vi "ERD Send Receive Example.vi"() -> ()   [LabVIEW 2016]
uses:
  type defs/ERD Read Data Out.ctl
  type defs/ERD Read Data In.ctl
  type defs/Data Type.ctl
  type defs/ERD Write Data In.ctl
  type defs/Source_Destination.ctl
  <vilib>/Utility/file.llb/Write To Spreadsheet File (string).vi
  library/GEA2_Toolkit.lvlib
panel:
  out "Continouous":T1[](array[typedef]) {"ERD Number" format="%.0x"}
  out "Raw Data Out":string
  in  "Write ERD List":T2[](array[typedef]) {"ERD Number" format="%.0x"}
  in  "Send ERD":bool
  in  "ERD to Read":T4[](array[typedef])=[{"ERD Number"=16499, "Data Type"=enum."string"}] {"ERD Number" format="%.0x"}
  out "Output Data Read":T1[](array[typedef]) {"ERD Number" format="%.0x"}
  in  "Read ERD":bool
  in  "Path":path
  in  "Board Index":i32
  in  "stop":bool
  # "HEWH Wifi Module\n0x600F - 01 Off\n0x600F - 00 On"
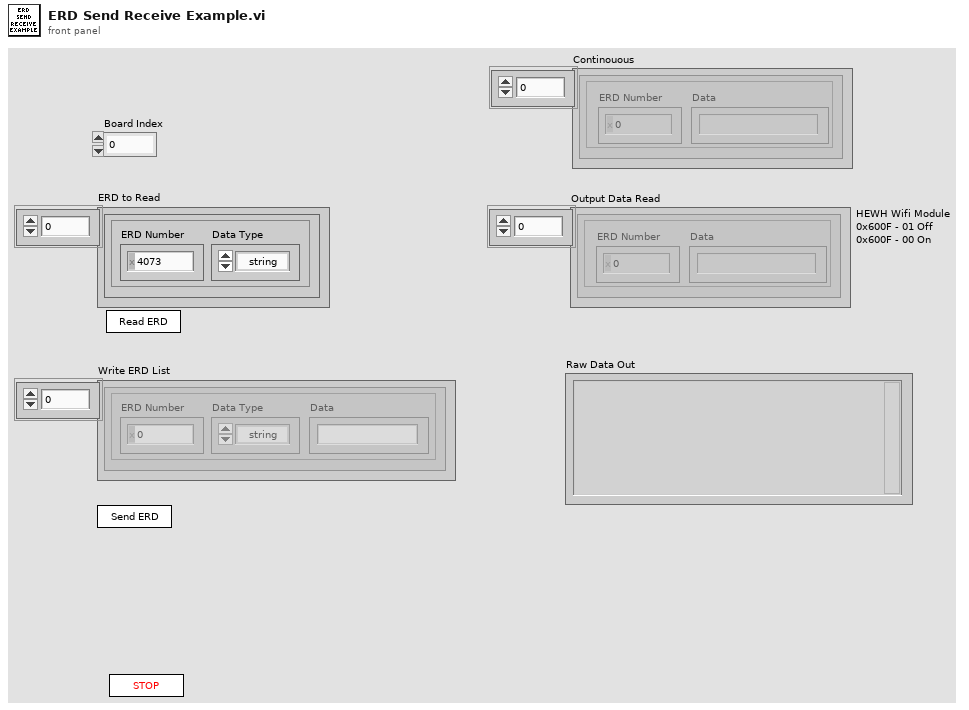
[diagram p1: front panel]
types:
  T1 = typedef "GEA2_Toolkit.lvlib/ERD Read Data Out.ctl" = cluster{"ERD Number":u16, "Data":string}
  T2 = typedef "GEA2_Toolkit.lvlib/ERD Write Data In.ctl" = cluster{"ERD Number":u16, "Data Type":T3, "Data":string}
  T3 = typedef "GEA2_Toolkit.lvlib/Data Type.ctl" = enum16{"string", "boolean", "uint8_t", "uint16_t", "uint32_t", "uint64_t"}
  T4 = typedef "GEA2_Toolkit.lvlib/ERD Read Data In.ctl" = cluster{"ERD Number":u16, "Data Type":T3}
  T5 = typedef "GEA2_Toolkit.lvlib/Source_Destination.ctl" = cluster{"Source":u8, "Destination":u8}
  T6 = enum32{"invalid app kind", "Development System", "Run Time System", "Student Edition", "Embedded LabVIEW", "Evaluation", "Custom"}
  T7 = enum32{"Invalid", "Standard", "Closed", "Hidden", "Minimized", "Maximized"}
  T8 = cluster{"Core":cluster{"Current VI Reference":refnum<vi>, "Close Panel on Exit?":bool}, "HEWH Appliance Data":string[][]}
  T9 = cluster{"Current VI Reference":refnum<vi>, "Close Panel on Exit?":bool}
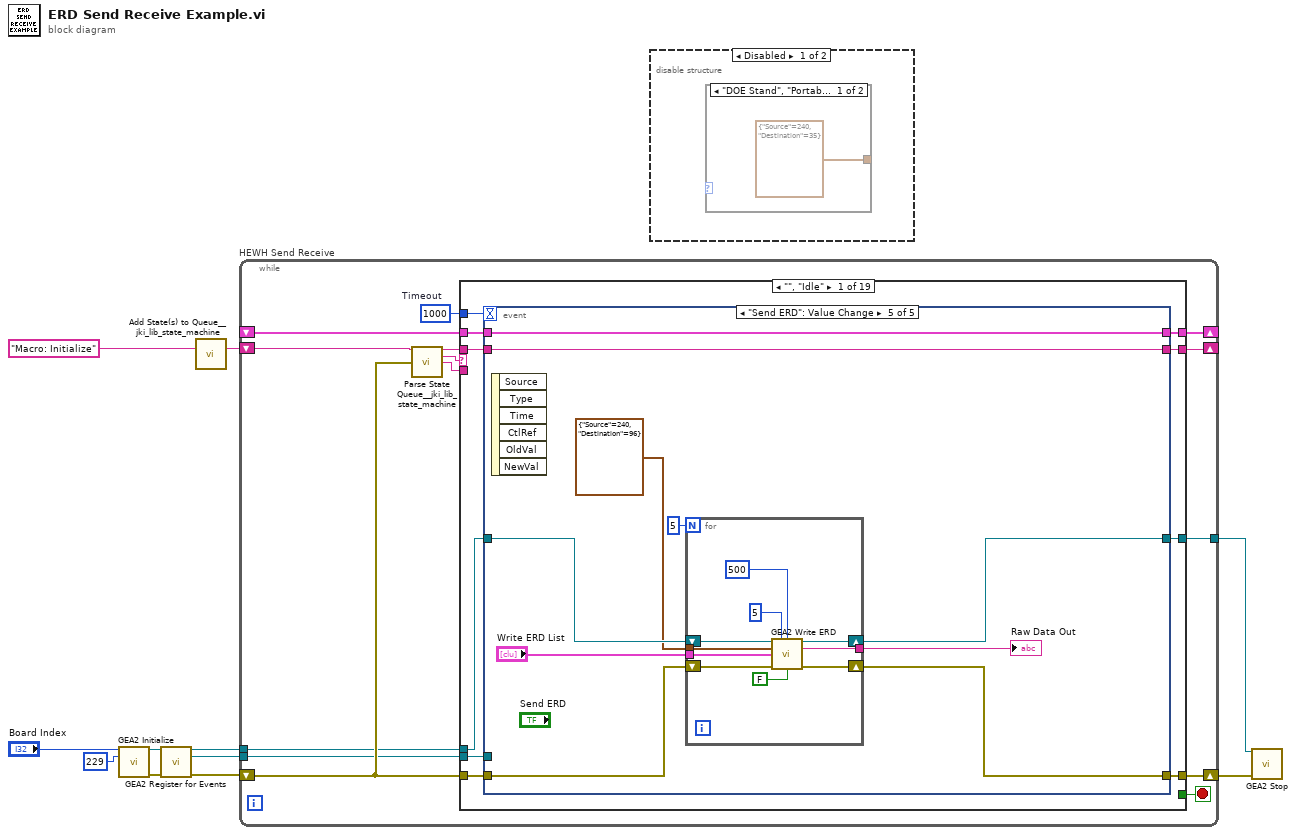
[diagram p0: block diagram]
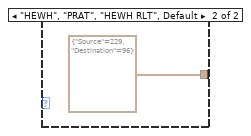
[diagram p2: hidden frame]
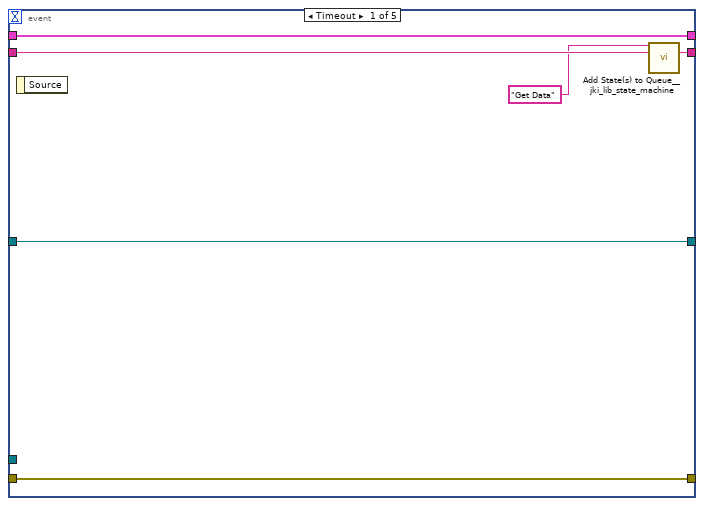
[diagram p4: hidden frame]
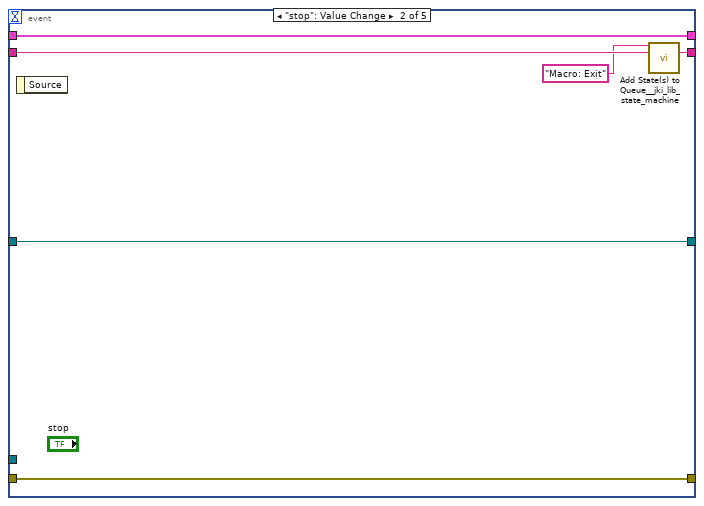
[diagram p5: hidden frame]
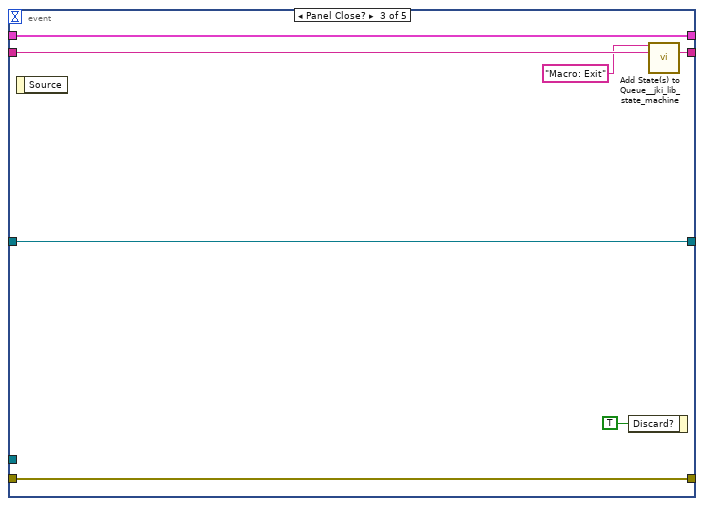
[diagram p6: hidden frame]
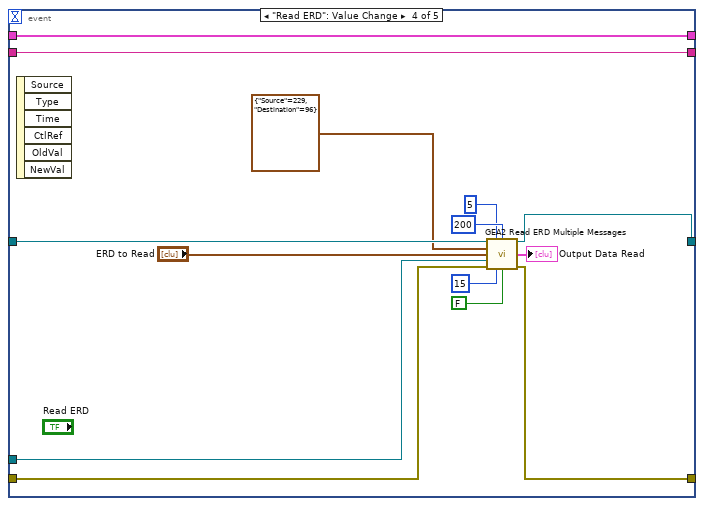
[diagram p7: hidden frame]
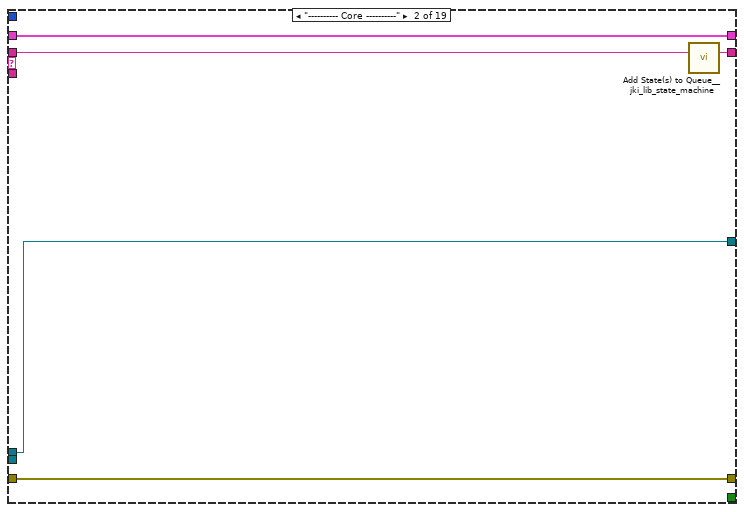
[diagram p8: hidden frame]
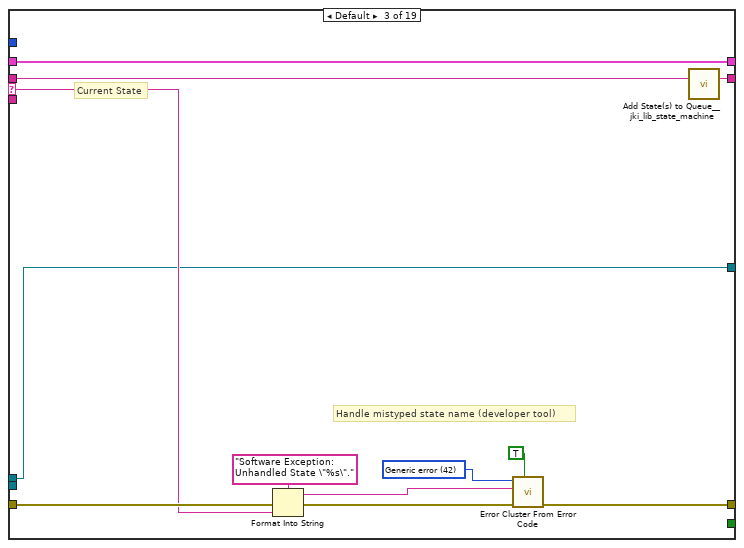
[diagram p9: hidden frame]
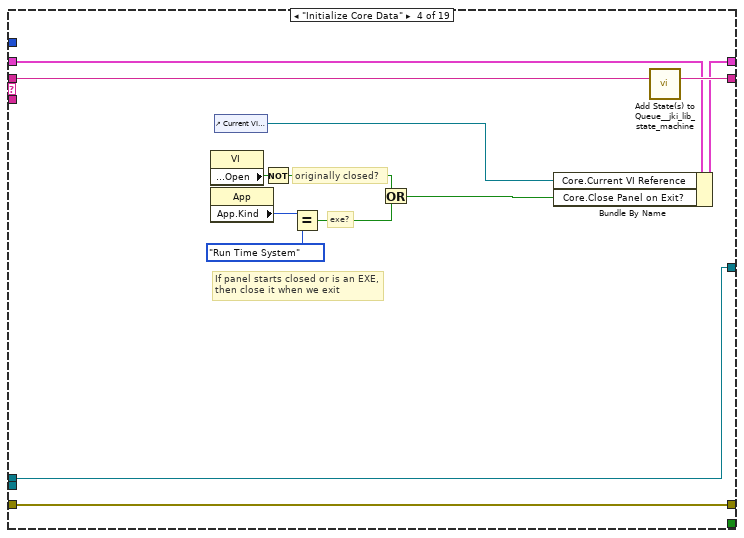
[diagram p10: hidden frame]
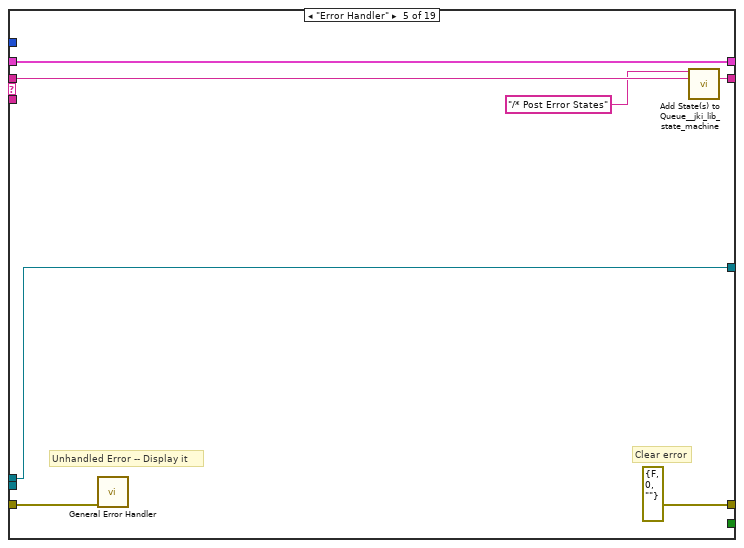
[diagram p11: hidden frame]
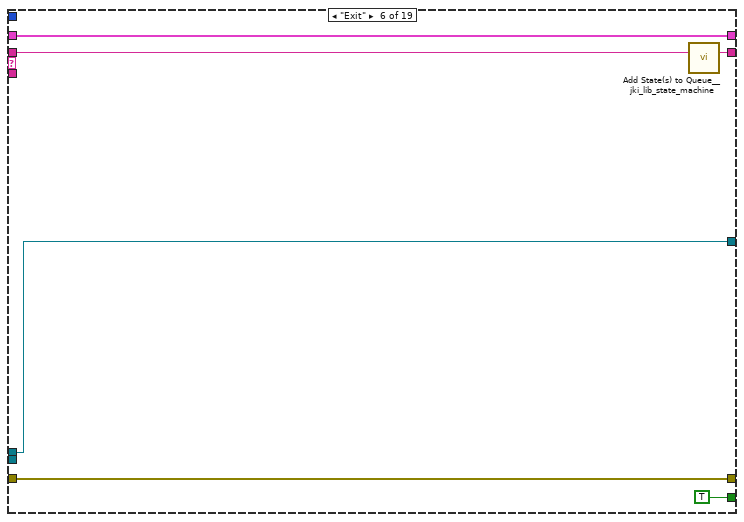
[diagram p12: hidden frame]
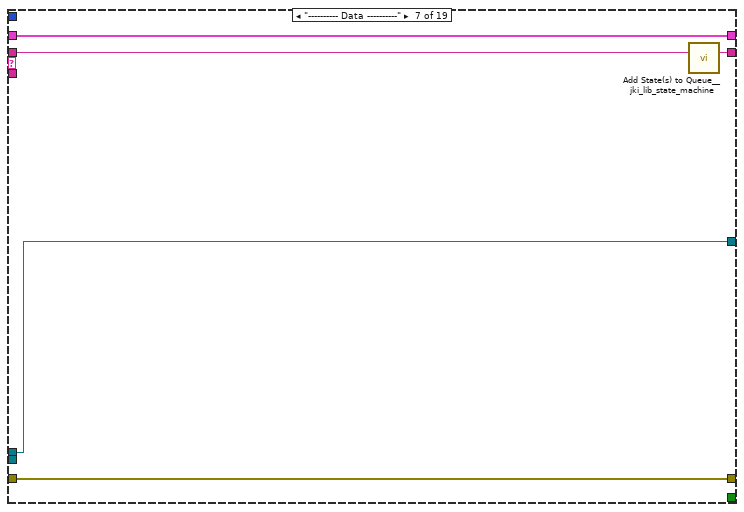
[diagram p13: hidden frame]
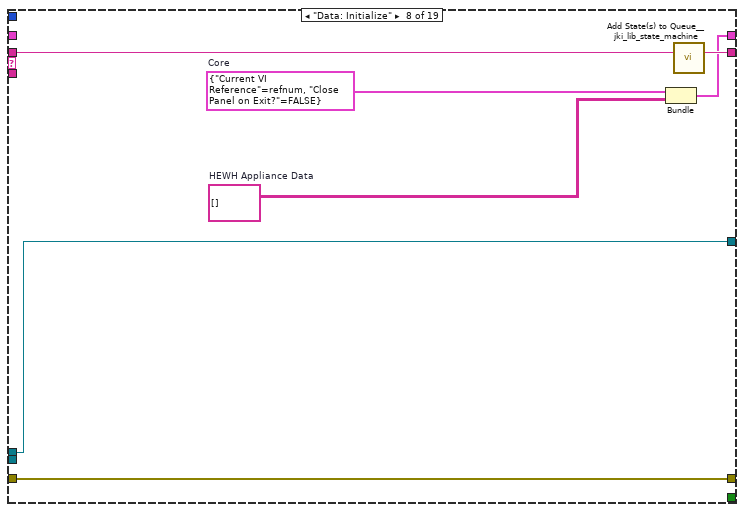
[diagram p14: hidden frame]
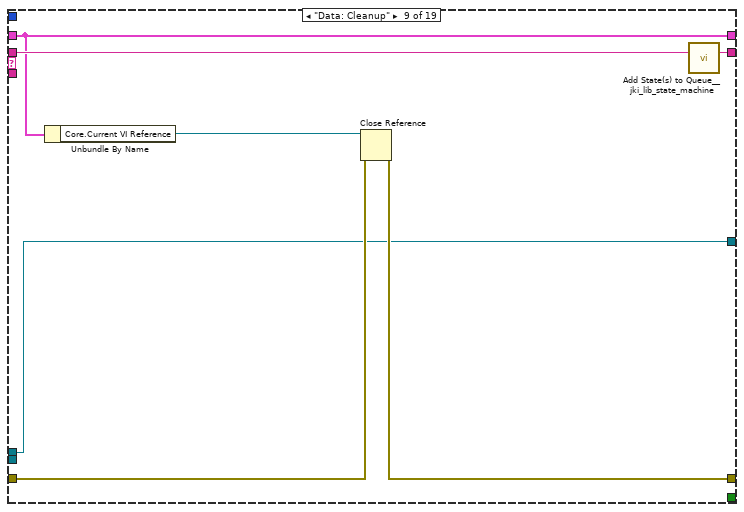
[diagram p15: hidden frame]
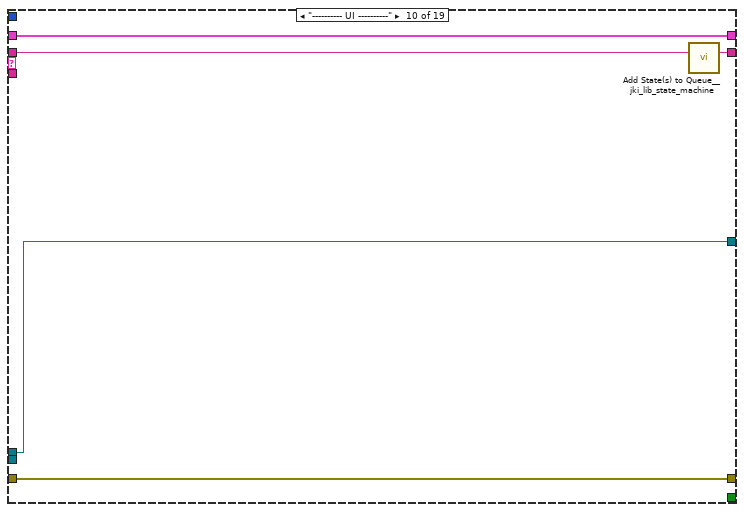
[diagram p16: hidden frame]
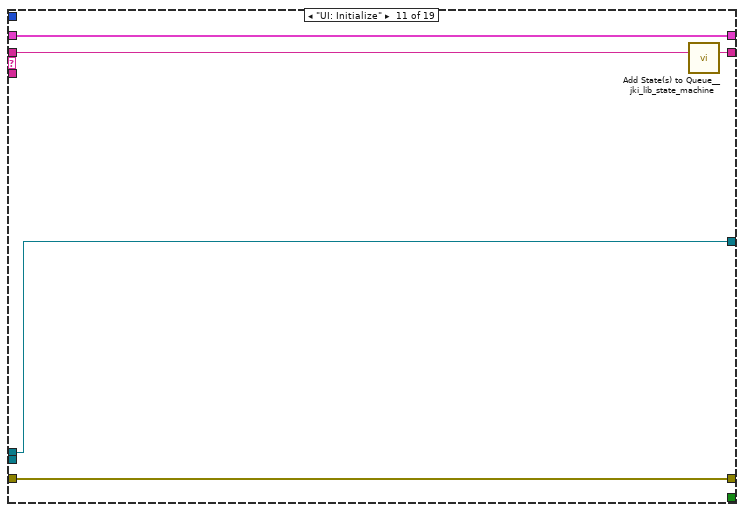
[diagram p17: hidden frame]
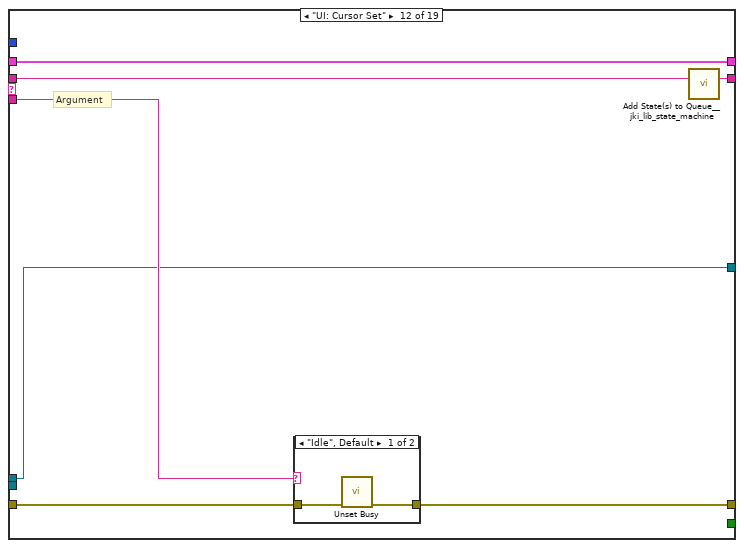
[diagram p18: hidden frame]
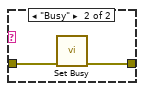
[diagram p19: hidden frame]
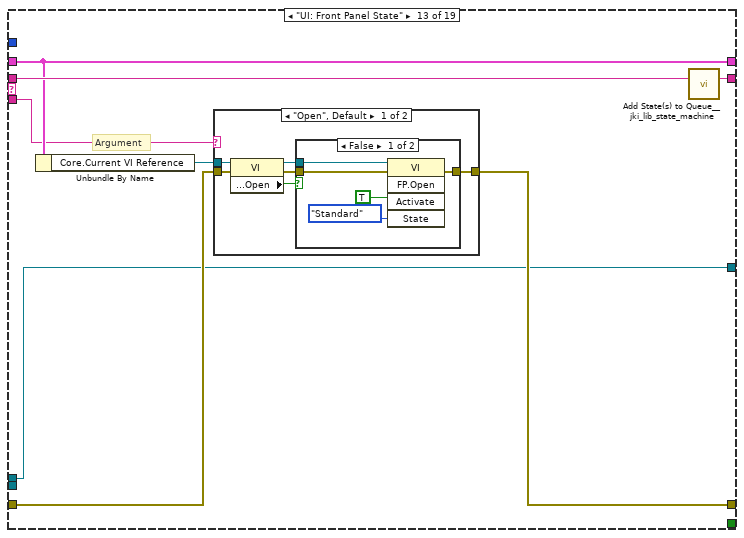
[diagram p20: hidden frame]
diagram:
  n1 = call "GEA2 Initialize.vi"("Board Index"="Board Index", "Source Address"=u8 229) -> ("GEA2 Reference Out"=w8:refnum<k24>, "error out"=w9:errorcluster)  [unwired: 11 in, 1 out]
  n2 = call "GEA2 Register for Events.vi"("GEA2 Reference In"=w8, "Error In"=w9) -> ("GEA2 Reference Out"=w3:refnum<k24>, "GEA2 Event Registration"=w2:refnum<event-registration>, "Error Out"=w5:errorcluster)  [unwired: 11 in]
  n3 = call <vilib>:"Add State(s) to Queue__jki_lib_state_machine.vi"("State(s) in (\"\")"="Macro: Initialize") -> ("States Out"=w7:string)  [unwired: 14 in]
  n4 = while "HEWH Send Receive" {
    shift-right: [w18] -> _
    shift-left: _ -> [w17]
    shift-right: [w21] -> w4
    shift-left: w5 -> [w15]
    shift-right: [w20] -> _
    shift-left: w7 -> [w22]
    tunnel: w3 -> [w14]
    tunnel: w2 -> [w13]
    tunnel: [w12] -> w1
    stop <- w19 stop-if-true
    w16 = 1000  # Timeout
    n5 = call <vilib>:"Parse State Queue__jki_lib_state_machine.vi"("State Queue"=w22, "Error In (no error)"=w15) -> ("Remaining States"=w24:string, "Current State"=w25:string, "Arguments"=w23:string)  [unwired: 11 in]
    n6 = case shown="\"\", \"Idle\"" w25 {
      selector: w25 -> [_ _ w95 _ _ _ _ _ _ _ _ _ _ _ _ _ _ _ _]
      tunnel: w24 -> [w35 w93 w99 w118 w125 w131 w136 w143 w150 w155 w160 w167 w179 w206 w212 w223 w228 w243 w252]
      tunnel: w23 -> [_ _ _ _ _ _ _ _ _ _ _ w162 w173 _ _ _ _ _ _]
      tunnel: w17 -> [w33 w90 w97 w109 w122 w129 w133 _ w145 w152 w158 w165 w175 w203 w209 w220 w225 w241 w247]
      tunnel: [w32 w91 w101 w115 errorcluster {"status"=FALSE, "code"=0, "source"=""} ("error out") w128 w134 w140 w146 w153 w157 w163 w176 w204 w210 w221 w226 w231 w248] -> w21
      tunnel: w15 -> [w31 w91 w100 w115 w121 w128 w134 w140 w147 w153 w157 w164 w177 w204 w210 w221 w226 w230 w249]
      tunnel: [w34 w92 w98 w117 w124 w130 w135 w142 w149 w154 w159 w166 w178 w205 w211 w222 w227 w242 w251] -> w20
      tunnel: [_ _ _ _ _ TRUE _ _ _ _ _ _ _ _ _ _ _ _ _] -> w19
      tunnel: [w30 w90 w97 w116 w122 w129 w133 w141 w145 w152 w158 w165 w175 w203 w209 w220 w225 w241 w247] -> w18
      tunnel: w16 -> [w29 _ _ _ _ _ _ _ _ _ _ _ _ _ _ _ _ _ _]
      tunnel: w14 -> [w28 w89 w94 w106 w119 w126 w132 w137 w144 w151 w156 w161 w172 w202 w207 w213 w224 w233 w245]
      tunnel: w13 -> [w27 _ _ _ _ _ _ _ _ _ _ _ _ _ _ _ _ w229 _]
      tunnel: [w26 w89 w94 w106 w119 w126 w132 w137 w144 w151 w156 w161 w172 w202 w207 w213 w224 w232 w245] -> w12
      frame "", "Idle" {
        n7 = event shown="[4] \"Send ERD\": Value Change" {
          selector: _ -> [_ _ _ _ _]
          dyn-events: _ -> [_ _ _ _ _]
          timeout: w29 -> [_ _ _ _ _]
          tunnel: w35 -> [w41 w47 w54 w67 w77]
          tunnel: [w40 w46 w53 w67 w77] -> w34
          tunnel: w33 -> [w38 w44 w51 w68 w78]
          tunnel: [w39 w45 w52 w56 w70] -> w32
          tunnel: w31 -> [w39 w45 w52 w57 w71]
          tunnel: [w38 w44 w51 w68 w78] -> w30
          tunnel: w28 -> [w37 w42 w48 w61 w76]
          tunnel: w27 -> [_ _ _ w60 _]
          tunnel: [w37 w42 w48 w58 w75] -> w26
          event Timeout {
            n8 = event-data() -> ()  [unwired: 1 in, 1 out]
            n9 = call <vilib>:"Add State(s) to Queue__jki_lib_state_machine.vi"("State(s) in Front (\"\")"="Get Data" ("State(s) in Front (\"\")"), "State(s) in (\"\")"=w41) -> ("States Out"=w40:string)  [unwired: 13 in]
          }
          event "stop": Value Change {
            n10 = event-data() -> ()  [unwired: 1 in, 1 out]
            n11 = call <vilib>:"Add State(s) to Queue__jki_lib_state_machine.vi"("State(s) in Front (\"\")"="Macro: Exit", "State(s) in (\"\")"=w47) -> ("States Out"=w46:string)  [unwired: 13 in]
          }
          event Panel Close? {
            n12 = event-data() -> ()  [unwired: 1 in, 1 out]
            n13 = event-data("Discard?"=TRUE) -> ()  [unwired: 1 in, 1 out]
            n14 = call <vilib>:"Add State(s) to Queue__jki_lib_state_machine.vi"("State(s) in Front (\"\")"="Macro: Exit", "State(s) in (\"\")"=w54) -> ("States Out"=w53:string)  [unwired: 13 in]
          }
          event "Read ERD": Value Change {
            n15 = event-data() -> ()  [unwired: 1 in, 6 out]
            n16 = call "GEA2 Read ERD Multiple Messages.vi"("GEA2 Reference In"=w61, "Retry Count"=5, "Read Timeout (ms)"=u32 200, "GEA Inputs"=T5 {"Source"=229, "Destination"=96}, "Read ERD List"="ERD to Read", "GEA2 Event Registration"=w60, "Error In"=w57, "#ERDs per message"=15, "Verify ERD Response?"=FALSE) -> ("GEA2 Reference Out"=w58:refnum<k24>, "ERD Data Out"=→"Output Data Read":T1[], "Error Out"=w56:errorcluster)  [unwired: 2 in, 2 out]
          }
          event "Send ERD": Value Change {
            n17 = event-data() -> ()  [unwired: 1 in, 6 out]
            n18 = for {
              N: 5 -> [_]
              tunnel: T5 {"Source"=240, "Destination"=96} ("GEA Inputs") -> [w86]
              tunnel: "Write ERD List" -> [w85]
              tunnel: [w81] -> w72
              shift-right: [w87] -> w75
              shift-left: w76 -> [w88]
              shift-right: [w79] -> w70
              shift-left: w71 -> [w80]
              n19 = call "GEA2 Write ERD.vi"("GEA2 Reference In"=w88, "Retry Count"=5, "Read Timeout (ms)"=u32 500, "GEA Inputs"=w86, "Write ERD List"=w85, "Error In"=w80, "Verify ERD Response?"=FALSE) -> ("GEA2 Reference Out"=w87:refnum<k24>, "Raw Data Out"=w81:string, "Error Out"=w79:errorcluster)  [unwired: 6 in]
            }
            "Raw Data Out" <- w72
          }
        }
      }
      frame "---------- Core ----------" {
        n20 = call <vilib>:"Add State(s) to Queue__jki_lib_state_machine.vi"("State(s) in (\"\")"=w93) -> ("States Out"=w92:string)  [unwired: 14 in]
      }
      frame Default {
        w104 = 42 items=["No error", "Argument error", "Memory is full", "Out of zone", "End of file", "File already open", "Generic file I/O error", "File not found", "File permission error", "Disk is full", "Duplicate path", "Too many files open", "System feature not enabled", "Resource file not found", "Cannot add resource", "Resource not found", "Image not found", "Image memory error", "Pen does not exist", "Config type invalid", "Config token not found", "Config parse error", "Config memory error", "Bad external code format", "Bad external code offset", "External code not present", "Null window", "Destroy window error", "Null menu", "Print aborted", "Bad print record", "Print driver error", "Windows error during printing", "Memory error during printing", "Print dialog error", "Generic print error", "Invalid device refnum", "Device not found", "Device parameter error", "Device unit error", "Cannot open device", "Device call aborted", "Generic error", "Cancelled by user", "Object ID too low", "Object ID too high", "Object not in heap", "Unknown heap", "Unknown object (invalid DefProc)", "Unknown object (DefProc not in table)", "Message out of range", "Invalid (null) method", "Unknown message", "Manager call not supported", "Bad address", "Network operation in progress", "Network operation timed out", "Connection is busy", "Network attribute not supported", "Network error", "Address in use", "System out of memory", "Connection aborted", "Connection refused", "Not connected", "Already connected", "Connection closed", "Initialization error (interapplication manager)", "Bad occurrence", "Wait on unbound occurrence handler", "Occurrence queue overflow", "Datalog type conflict", "Unused", "Unrecognized type (interapplication manager)", "Memory corrupt", "Failed to make temporary DLL", "Old CIN version", "Drag socket not found", "Failed to load drop-object", "Failed to register OLE object", "Failed to release OLE object", "Format specifier type mismatch", "Unknown format specifier", "Too few format specifiers", "Too many format specifiers", "Scan failed", "Newer CIN version", "Error converting to variant", "Runtime menu error", "Password tampered", "Variant attribute not found", "Incompatible variant data type", "Event data is not available", "Event Store is not present", "Occurrence is not found", "Event Queue is not created", "Event info is not available", "Refnum passed is NULL", "Error retrieving Class GUID", "Error retrieving CoClass GUID", "Error retrieving TypeLib GUID.", "Bad built application magic bytes.", "Specific driver is different from the specific driver associated with the Logical Name.", "There is no session opened to the class driver.", "Max Error", "MAX - Error with config objects", "MAX - Error loading configuration", "MAX - Group not supported"]
        # "Current State"
        # "Handle mistyped state name (developer tool)"
        n21 = Format Into String(format string="Software Exception: Unhandled State \"%s\"." ("message"), error in=w100, w95) -> (resulting string=w103:string, error out=w102:errorcluster)  [unwired: 1 in]
        n22 = call <vilib>:"Error Cluster From Error Code.vi"("show call chain? (False)"=TRUE, "error in (no error)"=w102, "error message (\"\")"=w103, "error code (0)"=w104) -> ("error out"=w101:errorcluster)  [unwired: 5 in]
        n23 = call <vilib>:"Add State(s) to Queue__jki_lib_state_machine.vi"("State(s) in (\"\")"=w99) -> ("States Out"=w98:string)  [unwired: 14 in]
      }
      frame "Initialize Core Data" {
        # "originally closed?"
        # "exe?"
        # "If panel starts closed or is an EXE, then close it when we exit"
        n24 = property class="VI"() -> ("Front Panel.Open"=w114:bool)  [unwired: 2 in, 2 out]
        n25 = property class="App"() -> ("App.Kind"=w113:T6)  [unwired: 2 in, 2 out]
        n26 = control-ref of="Current VI Reference"() -> (w107:refnum<vi>)
        n27 = Not(x=w114) -> (.not. x?=w111:bool)
        n28 = Equal?(x=w113, y=T6."Run Time System" ("Application:Kind")) -> (x = y?=w110:bool)
        n29 = Or(x=w111, y=w110) -> (x .or. y?=w108:bool)
        n30 = Bundle By Name(cluster=w109, "Core.Current VI Reference"=w107, "Core.Close Panel on Exit?"=w108) -> (w116:T8)
        n31 = call <vilib>:"Add State(s) to Queue__jki_lib_state_machine.vi"("State(s) in (\"\")"=w118) -> ("States Out"=w117:string)  [unwired: 14 in]
      }
      frame "Error Handler" {
        # "Unhandled Error -- Display it"
        # "Clear error"
        n32 = call <vilib>:"General Error Handler.vi"("error in (no error)"=w121) -> ()  [unwired: 10 in, 5 out]
        n33 = call <vilib>:"Add State(s) to Queue__jki_lib_state_machine.vi"("State(s) in Front (\"\")"="/* Post Error States", "State(s) in (\"\")"=w125) -> ("States Out"=w124:string)  [unwired: 13 in]
      }
      frame "Exit" {
        n34 = call <vilib>:"Add State(s) to Queue__jki_lib_state_machine.vi"("State(s) in (\"\")"=w131) -> ("States Out"=w130:string)  [unwired: 14 in]
      }
      frame "---------- Data ----------" {
        n35 = call <vilib>:"Add State(s) to Queue__jki_lib_state_machine.vi"("State(s) in (\"\")"=w136) -> ("States Out"=w135:string)  [unwired: 14 in]
      }
      frame "Data: Initialize" {
        w138 = string[][] []  # HEWH Appliance Data
        w139 = T9 {"Current VI Reference"=refnum, "Close Panel on Exit?"=FALSE}  # Core
        n36 = Bundle("Core"=w139, "HEWH Appliance Data"=w138) -> (w141:T8)  [unwired: 1 in]
        n37 = call <vilib>:"Add State(s) to Queue__jki_lib_state_machine.vi"("State(s) in (\"\")"=w143) -> ("States Out"=w142:string)  [unwired: 14 in]
      }
      frame "Data: Cleanup" {
        n38 = Unbundle By Name(w145) -> ("Core.Current VI Reference"=w148:refnum<vi>)
        n39 = Close Reference(reference=w148, error in (no error)=w147) -> (error out=w146:errorcluster)
        n40 = call <vilib>:"Add State(s) to Queue__jki_lib_state_machine.vi"("State(s) in (\"\")"=w150) -> ("States Out"=w149:string)  [unwired: 14 in]
      }
      frame "---------- UI ----------" {
        n41 = call <vilib>:"Add State(s) to Queue__jki_lib_state_machine.vi"("State(s) in (\"\")"=w155) -> ("States Out"=w154:string)  [unwired: 14 in]
      }
      frame "UI: Initialize" {
        n42 = call <vilib>:"Add State(s) to Queue__jki_lib_state_machine.vi"("State(s) in (\"\")"=w160) -> ("States Out"=w159:string)  [unwired: 14 in]
      }
      frame "UI: Cursor Set" {
        # "Argument"
        n43 = case shown="\"Idle\", Default" w162 {
          tunnel: w164 -> [w169 w171]
          tunnel: [w168 w170] -> w163
          frame "Idle", Default {
            n44 = call <vilib>:"Unset Busy.vi"("error in (no error)"=w169) -> ("error out"=w168:errorcluster)  [unwired: 10 in]
          }
          frame "Busy" {
            n45 = call <vilib>:"Set Busy.vi"("error in (no error)"=w171) -> ("error out"=w170:errorcluster)  [unwired: 9 in, 1 out]
          }
        }
        n46 = call <vilib>:"Add State(s) to Queue__jki_lib_state_machine.vi"("State(s) in (\"\")"=w167) -> ("States Out"=w166:string)  [unwired: 14 in]
      }
      frame "UI: Front Panel State" {
        # "Argument"
        n47 = Unbundle By Name(w175) -> ("Core.Current VI Reference"=w174:refnum<vi>)
        n48 = case shown="\"Open\", Default" w173 {
          tunnel: w177 -> [w183 w196]
          tunnel: [w185 w197] -> w176
          tunnel: w174 -> [w184 w194]
          frame "Open", Default {
            n49 = property class="VI"(reference=w184, error in=w183) -> (reference out=w181:refnum<vi>, error out=w182:errorcluster, "Front Panel.Open"=w180:bool)
            n50 = case shown="False" w180 {
              tunnel: [w188 w191] -> w185
              tunnel: w182 -> [w187 w191]
              tunnel: w181 -> [w186 _]
              frame False {
                n51 = invoke class="VI" method="FP.Open"(reference=w186, error in=w187, "Activate"=TRUE, "State"=T7."Standard") -> (error out=w188:errorcluster)  [unwired: 1 in, 4 out]
              }
              frame True {
              }
            }
          }
          frame "Close" {
            n52 = property class="VI"(reference=w194, error in=w196) -> (reference out=w193:refnum<vi>, error out=w195:errorcluster, "Front Panel.Open"=w192:bool)
            n53 = case shown="True" w192 {
              tunnel: [w198 w201] -> w197
              tunnel: w195 -> [w198 w200]
              tunnel: w193 -> [_ w199]
              frame False {
              }
              frame True {
                n54 = invoke class="VI" method="FP.Close"(reference=w199, error in=w200) -> (error out=w201:errorcluster)  [unwired: 1 in, 2 out]
              }
            }
          }
        }
        n55 = call <vilib>:"Add State(s) to Queue__jki_lib_state_machine.vi"("State(s) in (\"\")"=w179) -> ("States Out"=w178:string)  [unwired: 14 in]
      }
      frame "---------- Macro ----------" {
        n56 = call <vilib>:"Add State(s) to Queue__jki_lib_state_machine.vi"("State(s) in (\"\")"=w206) -> ("States Out"=w205:string)  [unwired: 14 in]
      }
      frame "Macro: Initialize" {
        w208 = "Data: Initialize\nInitialize Core Data\nUI: Initialize\nUI: Front Panel State >> Open"  # Data: Initialize Initialize Core Data UI: Initialize UI: Front Panel State >> Open
        n57 = call <vilib>:"Add State(s) to Queue__jki_lib_state_machine.vi"("State(s) in Front (\"\")"=w208, "State(s) in (\"\")"=w212) -> ("States Out"=w211:string)  [unwired: 13 in]
      }
      frame "Macro: Exit" {
        n58 = Unbundle By Name(w220) -> ("Core.Close Panel on Exit?"=w219:bool)
        n59 = Select(t="UI: Front Panel State >> Close", s=w219, f="") -> (s? t:f=w216:string)
        n60 = call <vilib>:"Add State(s) to Queue__jki_lib_state_machine.vi"("State(s) in (\"\")"=w216, "State(s) at Back (\"\")"="Data: Cleanup\nExit") -> ("States Out"=w214:string)  [unwired: 13 in]
        n61 = call <vilib>:"Add State(s) to Queue__jki_lib_state_machine.vi"("State(s) in Front (\"\")"=w214, "State(s) in (\"\")"=w223) -> ("States Out"=w222:string)  [unwired: 13 in]
      }
      frame "---------- New Category ----------" {
        n62 = call <vilib>:"Add State(s) to Queue__jki_lib_state_machine.vi"("State(s) in (\"\")"=w228) -> ("States Out"=w227:string)  [unwired: 14 in]
      }
      frame "Get Data" {
        n63 = local read "ERD to Read"() -> (w234:T4[])
        n64 = call "GEA2 Read ERD Multiple Messages.vi"("GEA2 Reference In"=w233, "Retry Count"=5, "Read Timeout (ms)"=u32 200, "GEA Inputs"=T5 {"Source"=229, "Destination"=96}, "Read ERD List"=w234, "GEA2 Event Registration"=w229, "Error In"=w230, "#ERDs per message"=15, "Verify ERD Response?"=FALSE) -> ("GEA2 Reference Out"=w232:refnum<k24>, "ERD Data Out"=→"Continouous":T1[], "Error Out"=w231:errorcluster)  [unwired: 2 in, 2 out]
        n65 = call <vilib>:"Add State(s) to Queue__jki_lib_state_machine.vi"("State(s) in (\"\")"=w243) -> ("States Out"=w242:string)  [unwired: 14 in]
      }
      frame "Save Data" {
        n66 = Unbundle By Name(w247) -> ("HEWH Appliance Data"=w246:string[][])
        n67 = First Call?() -> (First Call?: T/F=w250:bool)
        n68 = case shown="False" w250 {
          tunnel: "Path" -> [w256 w264]
          tunnel: w246 -> [w259 w262]
          tunnel: w249 -> [w253 w260]
          tunnel: [w253 w260] -> w248
          frame False {
            n69 = Index Array(array=w259, index (col)=1 ("disabled index (col)")) -> (element=w257:string[])  [unwired: 1 in]
            n70 = call-poly <vilib>:"Write To Spreadsheet File.vi"("delimiter (\\t)"="," ("delimiter (\\t)"), "append to file? (new file:F)"=TRUE, "1D data"=w257, "file path (dialog if empty)"=w256) -> ()  [unwired: 4 in, 1 out]
          }
          frame True {
            n71 = Transpose 2D Array(2D array=w262) -> (transposed array=w261:string[][])
            n72 = call-poly <vilib>:"Write To Spreadsheet File.vi"("delimiter (\\t)"="," ("delimiter (\\t)"), "2D data"=w261, "file path (dialog if empty)"=w264) -> ()  [unwired: 5 in, 1 out]
          }
        }
        n73 = call <vilib>:"Add State(s) to Queue__jki_lib_state_machine.vi"("State(s) in (\"\")"=w252) -> ("States Out"=w251:string)  [unwired: 14 in]
      }
    }
  }
  n74 = disable-structure shown="Disabled" {
    frame Disabled {
      n75 = case shown="\"DOE Stand\", \"Portable Stand\", \"HCC\"" {
        selector: _ -> [_ _]
        tunnel: [T5 {"Source"=240, "Destination"=35} ("GEA Inputs") T5 {"Source"=229, "Destination"=96} ("GEA Inputs")] -> _
        frame "DOE Stand", "Portable Stand", "HCC" {
        }
        frame "HEWH", "PRAT", "HEWH RLT", Default {
        }
      }
    }
    frame Enabled {
    }
  }
  n76 = call "GEA2 Stop.vi"("GEA2 Reference Out"=w1, "Error In"=w4) -> ()  [unwired: 13 in, 1 out]
